vi "ThermoCouple_Read.vi"(0 "task":refnum<k21>, 5 "samples":i32=-1, 7 "period (ms)":i32, 9 "prev Temps":dbl[](array[numeric]), 11 "error in":errorcluster) -> (4 "dt":dbl, 6 "Temps":dbl[](array[numeric]), 8 "Gradients":dbl[](array[numeric]), 15 "error out":errorcluster)   [LabVIEW 2024]
uses:
  <vilib>/DAQmx/read.llb/DAQmx Read (Analog 2D DBL NChan NSamp).vi
  <vilib>/DAQmx/miscellaneous.llb/DAQmx Fill In Error Info.vi
  <vilib>/Analysis/NI_AALBase.lvlib
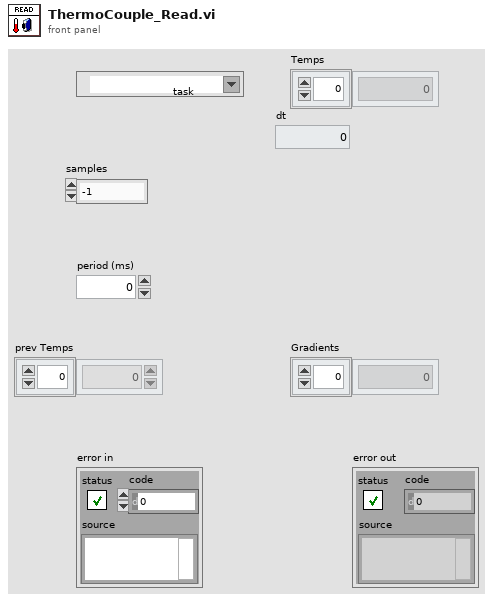
[diagram p1: front panel]
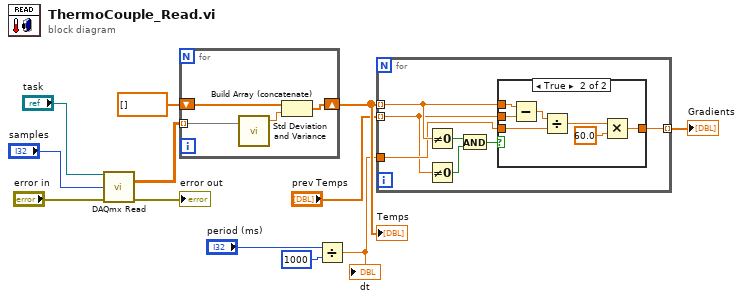
[diagram p0: block diagram]
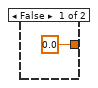
[diagram p2: hidden frame]
diagram:
  n1 = call-poly <vilib>:"DAQmx Read.vi"("task/channels in"="task", "number of samples per channel"="samples", "error in"="error in") -> ("data"=w12:dbl[][], "error out"=→"error out":errorcluster)  [unwired: 10 in, 1 out]
  n2 = for {
    tunnel: w12 -> [w14] mode=indexing
    shift-right: [w16] -> w7
    shift-left: dbl[] [] -> [w15]
    n3 = call <vilib>:"Std Deviation and Variance.vi"("X"=w14) -> ("mean"=w13:dbl)  [unwired: 1 in, 2 out]
    n4 = Build Array (concatenate)(w15, w13) -> (w16:dbl[])
  }
  "Temps" <- w7
  n5 = Divide(x="period (ms)", y=1000) -> (x/y=w4:dbl)
  "dt" <- w4
  n6 = for {
    tunnel: w7 -> [w21] mode=indexing
    tunnel: "prev Temps" -> [w17] mode=indexing
    tunnel: w4 -> [w19]
    tunnel: [w18] -> w2 mode=indexing
    n7 = Not Equal To 0?(x=w21) -> (x != 0?=w22:bool)
    n8 = Not Equal To 0?(x=w17) -> (x != 0?=w23:bool)
    n9 = And(x=w22, y=w23) -> (x .and. y?=w20:bool)
    n10 = case shown="True" w20 {
      tunnel: w21 -> [_ w31]
      tunnel: w17 -> [_ w30]
      tunnel: w19 -> [_ w26]
      tunnel: [0.0 w25] -> w18
      frame False {
      }
      frame True {
        n11 = Subtract(x=w31, y=w30) -> (x-y=w29:dbl)
        n12 = Divide(x=w29, y=w26) -> (x/y=w28:dbl)
        n13 = Multiply(x=w28, y=60.0) -> (x*y=w25:dbl)
      }
    }
  }
  "Gradients" <- w2
